vi "Actor Core.vi"(8 "error in":errorcluster, 11 "Controller in":refnum<class "Controller.lvclass">) -> (0 "error out":errorcluster, 3 "Actor out":refnum<class "Actor.lvclass">)   [LabVIEW 2020, in "Controller.lvlib" / "Controller.lvclass"]
doc: "(<B>Filename</B>: Actor Framework.lvlib:Actor.lvclass:Actor Core.vi)\n\nReceives messages to the actor, reacts to them, and initiates any error handling that may shut the actor down.\n\nDescendant classes may override this VI to append parallel tasks for the actor to complete while it handles messages. Overrides use the Call Parent Class Method node."
uses:
  Controller.lvclass
  <vilib>/ActorFramework/Actor/Actor.lvclass
  MVVM Framework/MVVM Abstruct Controller/MVVM Abstruct Controller/MVVM Abstruct Controller.lvclass
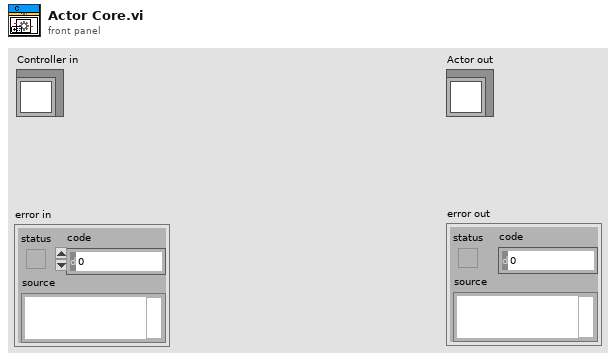
[diagram p1: front panel]
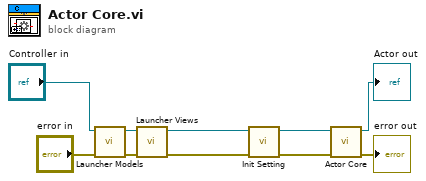
[diagram p0: block diagram]
diagram:
  n1 = call "Launcher Models.vi"("error in (no error)"="error in", "Controller in"="Controller in") -> ("error out"=w6:errorcluster, "Controller out"=w5:refnum<class "Controller.lvclass">)  [unwired: 8 in]
  n2 = call "Launcher Views.vi"("error in (no error)"=w6, "Controller in"=w5) -> ("error out"=w2:errorcluster, "Controller out"=w4:refnum<class "Controller.lvclass">)  [unwired: 8 in]
  n3 = call "Init Setting.vi"("error in (no error)"=w2, "Controller in"=w4) -> ("error out"=w1:errorcluster, "Controller out"=w3:refnum<class "Controller.lvclass">)  [unwired: 8 in]
  n4 = call-parent "Actor Core.vi"("error in"=w1, "Abstruct View in"=w3) -> ("error out"=→"error out":errorcluster, "Actor out"=→"Actor out":refnum<class "Actor.lvclass">)  [unwired: 8 in]
